vi "Generate Argument Type Info.vi"(8 "error in (no error)":errorcluster, 11 "Data Type":variant) -> (0 "error out":errorcluster, 3 "Array":T1[](array[typedef]))   [LabVIEW 2020, in "G-Embedded-Python-Interpreter-Toolkit.lvlib"]
uses:
  G-Embedded-Python-Interpreter-Toolkit.lvlib
  Type Information.ctl
  <vilib>/Utility/Data Type/Type Definitions/Data Type.ctl
  Python Object Reference.ctl
  Python Object Type.ctl
  Variant to Type Info.vi/8cdebbe9-3e59-4fbe-97b0-695fa0ebc24d.vi
  <vilib>/Utility/error.llb/Error Cluster From Error Code.vi
  <vilib>/Utility/Data Type/Get Array Information.vi
  <vilib>/Comparison/Equal/Equal Functor/Equal Functor.lvclass
  <vilib>/Utility/Data Type/NI_Data Type.lvlib
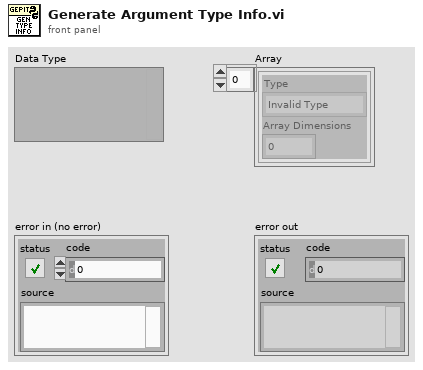
[diagram p1: front panel]
types:
  T1 = typedef "G-Embedded-Python-Interpreter-Toolkit.lvlib/Type Information.ctl" = cluster{"Type":T2, "Array Dimensions":u8}
  T2 = typedef "NI_Data Type.lvlib/Data Type.ctl" = enum8{"Invalid Type", "Void", "I8", "I16", "I32", "I64", "U8", "U16", "U32", "U64", "Single Float", "Double Float", "Extended Float", "Single Complex", "Double Complex", "Extended Complex", "Enum U8", "Enum U16", "Enum U32", "Enum U64", "Single Float With Unit", "Double Float With Unit", "Extended Float With Unit", "Single Complex with Unit", "Double Complex with Unit", "Extended Complex with Unit", "Boolean", "String", "Path", "Picture", "Tag", "Array", "Cluster", "Variant", "LV Variant", "Waveform", "Timestamp", "Digital Waveform", "Digital Data", "ExpressData", "Refnum", "External Data", "VI", "Poly VI", "LabVIEW Class Instance", "Fixed Point", "Set Collection", "Map Collection"}
  T3 = typedef "G-Embedded-Python-Interpreter-Toolkit.lvlib/Python Object Reference.ctl" = refnum<k1>
  T4 = typedef "NI_Data Type.lvlib/Type Definition Info.ctl" = cluster{"Name":string, "Timestamp":u32}
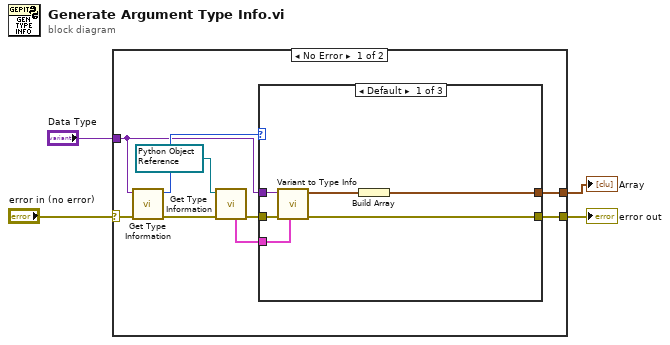
[diagram p0: block diagram]
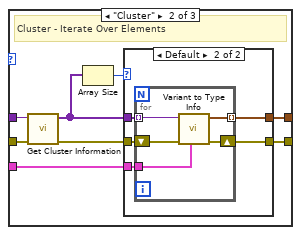
[diagram p2: hidden frame]
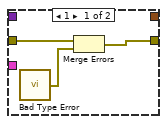
[diagram p3: hidden frame]
diagram:
  n1 = case shown="No Error" "error in (no error)" {
    selector: "error in (no error)" -> [w11 w42]
    tunnel: [w13 w42] -> w4
    tunnel: [w12 _] -> w3
    tunnel: "Data Type" -> [w8 _]
    frame No Error {
      w6 = T3 refnum items=["PyObj"] ("Python Object Refnum")
      n2 = call <vilib>:"Get Type Information.vi"("error in (no error)"=w11, "variant"=w8) -> ("error out"=w10:errorcluster, "type"=w9:T2)  [unwired: 5 in, 3 out]
      n3 = call <vilib>:"Get Type Information.vi"("error in (no error)"=w10, "variant"=w6) -> ("error out"=w7:errorcluster, "type definition info"=w5:T4)  [unwired: 5 in, 3 out]
      n4 = case shown="Default" w9 {
        tunnel: [w16 w27 w41] -> w13
        tunnel: [w14 w24 _] -> w12
        tunnel: w8 -> [w17 w25 _]
        tunnel: w7 -> [w19 w23 w41]
        tunnel: w5 -> [w18 w22 _]
        frame Default {
          n5 = call "Variant to Type Info.vi"("Py-Object Type Signature"=w18, "error in (no error)"=w19, "Type"=w17) -> ("error out"=w16:errorcluster, "Type Info"=w15:T1)  [unwired: 7 in]
          n6 = Build Array(w15) -> (w14:T1[])
        }
        frame "Cluster" {
          # "Cluster - Iterate Over Elements"
          n7 = call <vilib>:"Get Cluster Information.vi"("error in (no error)"=w23, "variant"=w25) -> ("error out"=w26:errorcluster, "cluster elements"=w21:variant[])  [unwired: 8 in]
          n8 = Array Size(array=w21) -> (size(s)=w20:i32)
          n9 = case shown="Default" w20 {
            tunnel: [w29 w35] -> w27
            tunnel: w26 -> [w30 w34]
            tunnel: [_ w33] -> w24
            tunnel: w22 -> [_ w32]
            tunnel: w21 -> [_ w31]
            frame 1 {
              n10 = call "Bad Type Error.vi"() -> ("Unsupported Type Error"=w28:errorcluster)
              n11 = Merge Errors(w30, w28) -> (w29:errorcluster)
            }
            frame Default {
              n12 = for {
                tunnel: w31 -> [w37] mode=indexing
                tunnel: [w40] -> w33 mode=indexing
                shift-right: [w38] -> w35
                shift-left: w34 -> [w39]
                tunnel: w32 -> [w36]
                n13 = call "Variant to Type Info.vi"("Py-Object Type Signature"=w36, "error in (no error)"=w39, "Type"=w37) -> ("error out"=w38:errorcluster, "Type Info"=w40:T1)  [unwired: 7 in]
              }
            }
          }
        }
        frame "Void" {
          # "Empty - No Arguments"
        }
      }
    }
    frame Error {
    }
  }
  "error out" <- w4
  "Array" <- w3
